vi "PH_ImageCalibrator.ProcCases.vi"(0 "i ref in":refnum<vi>, 1 "selector":string, 2 "data":T1, 3 "call cluster":T2={"Object"="", "Selector"="", "CallType"=enum."synchronous", "Async Object"="", "Async Selector"="", "Data Descriptor"="", "Data"=[], "Error #"=0, "Expire"=0}, 5 "error in":errorcluster) -> (14 "i ref out":refnum<vi>, 17 "answer cluster":T2={"Object"="", "Selector"="", "CallType"=enum."synchronous", "Async Object"="", "Async Selector"="", "Data Descriptor"="", "Data"=[], "Error #"=0, "Expire"=0}, 19 "error out":errorcluster)   [LabVIEW 2014, in "PH_ImageCalibrator.lvlib"]
doc: "This method is called by a process from within the default case in the event loop. The methods of a class that are linked to events will be called from THIS method. Add your code here."
uses:
  PH_ImageCalibrator.lvlib
  CSCore/CSSystem/CoreDefs/CoreDefs.call_type.ctl
  CSCore/BaseProcess/BaseProcess.descriptor string definition.ctl
  CSCore/CSSystem/CoreDefs/CoreDefs.rawDataType.ctl
  CSCore/CSSystem/CoreLib/CoreLib.string 2 byte array.vi
  CSCore/CSSystem/CoreLib/CoreLib.byte array 2 string.vi
  CSCore/BaseProcess/BaseProcess.lvlib
  CSCore/CSSystem/CoreLib/CoreLib.lvlib
  CSCore/BaseSM/BaseSM.lvlib
  PH_Img_BaseClass/PH_Img_BaseClass.lvlib
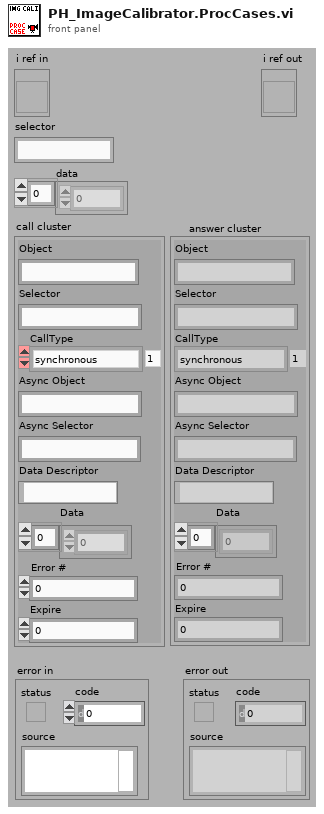
[diagram p1: front panel]
types:
  T1 = typedef "CoreDefs.rawDataType.ctl" = i8[]
  T2 = typedef "CoreDefs.call_type.ctl" = cluster{"Object":string, "Selector":string, "CallType":enum16{"simple", "synchronous", "asynchronous"}, "Async Object":string, "Async Selector":string, "Data Descriptor":T3, "Data":T1, "Error #":i32, "Expire":u32}
  T3 = typedef "BaseProcess.lvlib/BaseProcess.descriptor string definition.ctl" = string
  T4 = typedef "PH_ImageCalibrator.lvlib/PH_ImageCalibrator.i attribute.ctl" = cluster{"GUI Refs":cluster{"Available Cams":refnum<vi>, "OK":refnum<vi>, "Skip":refnum<vi>, "Repeat":refnum<vi>, "Cancel":refnum<vi>, "Length [mm]":refnum<vi>, "Energy [mJ]":refnum<vi>, "Dialog":refnum<vi>}, "Cam instances":string[], "Dark Pics":cluster{"#":i32, "BI taken":bool}, "Lin Cali":cluster{"Distance [Pixel]":dbl, "Distance [mm]":dbl, "Lin Cali Factor [mm/Pixel]":dbl}, "Energy Cali":cluster{"Pixelsum":dbl, "Energy [mJ]":dbl, "Energy Cali factor [mJ/Pixelsum]":dbl, "Underground subtracted?":bool, "#":i32}, "Images":cluster{"Background":T5, "Energy":T5}}
  T5 = typedef "IMAQ Image.ctl" = refnum<image>
  T6 = typedef "PH_Img_BaseClass.lvlib/PH_Img_BaseClass.i attribute.ctl" = cluster{"GUI Refs":T7, "Timeout Image [ms]":i32, "Default Periodic Period [ms]":i32, "Camera":cluster{"Instancename":string, "Notifier":refnum<notifier>}, "Palette":T8, "Cam Settings":cluster{"Cam ID":string, "Gain":dbl, "Brightness":dbl, "Shutter":dbl, "Cam Info Failure":bool, "Mode":i32}}
  T7 = typedef "PH_Img_BaseClass.lvlib/PH_Img_BaseClass.GUI Refs.ctl" = cluster{"Timeout":refnum<vi>, "Image":refnum<vi>, "Palette":refnum<vi>, "Timeout Set":refnum<vi>}
  T8 = typedef "PH_Img_BaseClass.lvlib/PH_Img_BaseClass.Palette.ctl" = i32
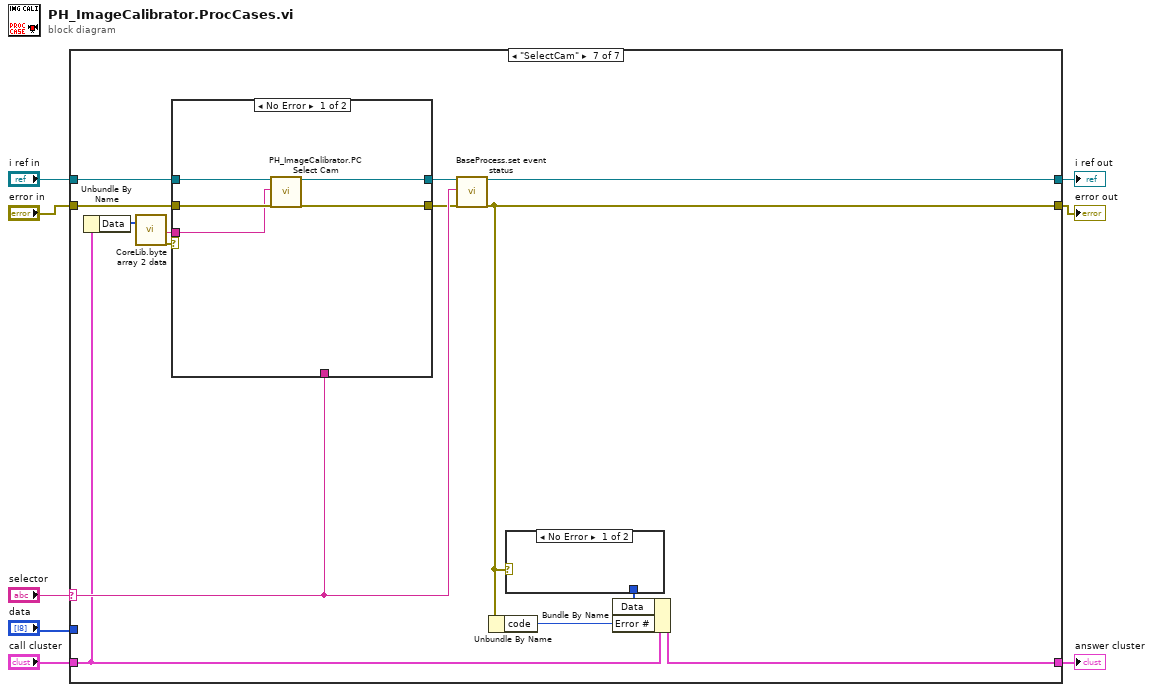
[diagram p0: block diagram]
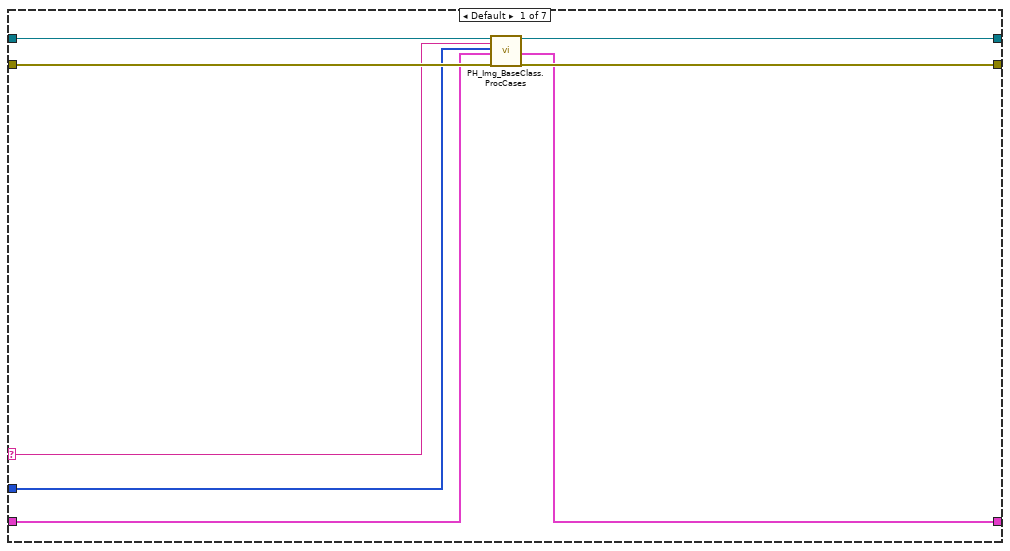
[diagram p2: hidden frame]
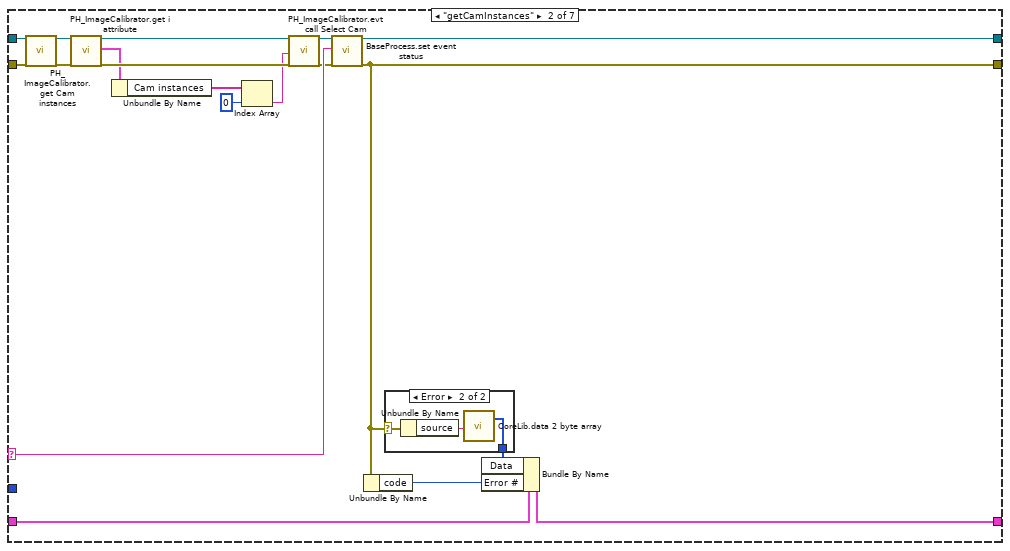
[diagram p3: hidden frame]
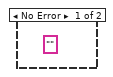
[diagram p4: hidden frame]
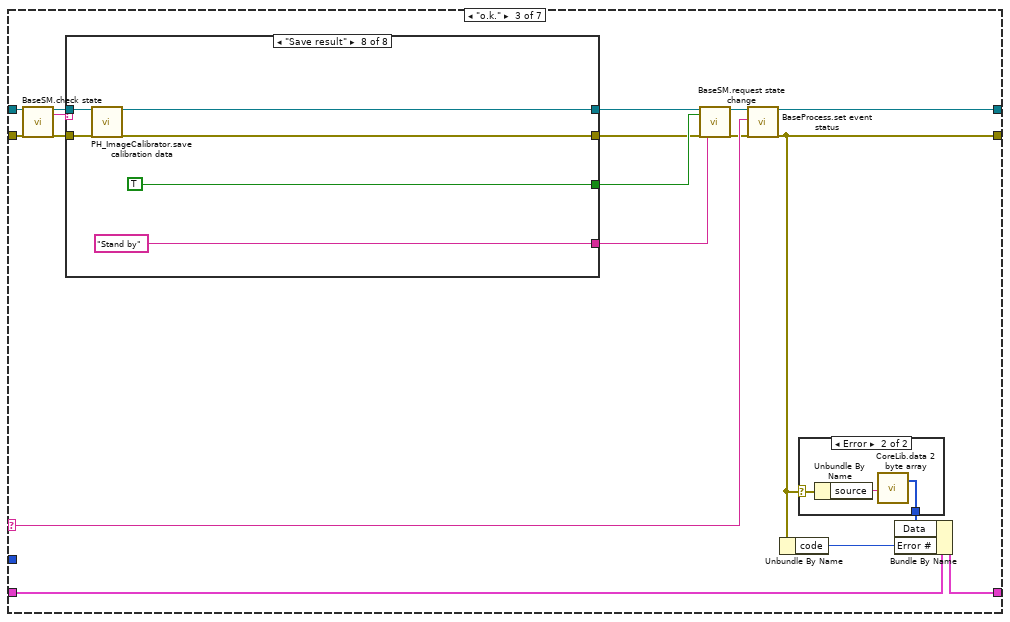
[diagram p5: hidden frame]
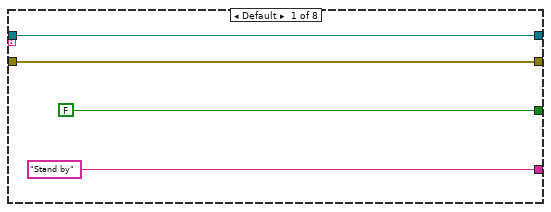
[diagram p6: hidden frame]
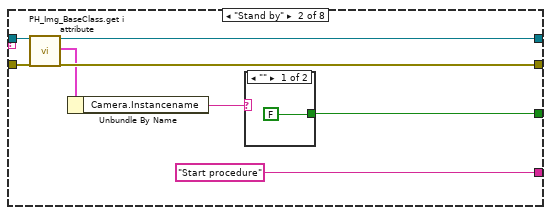
[diagram p7: hidden frame]
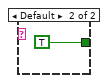
[diagram p8: hidden frame]
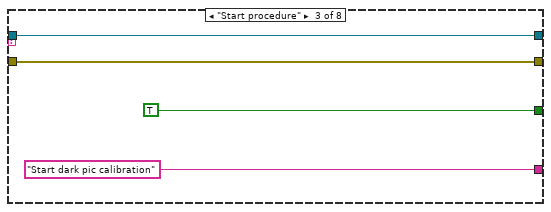
[diagram p9: hidden frame]
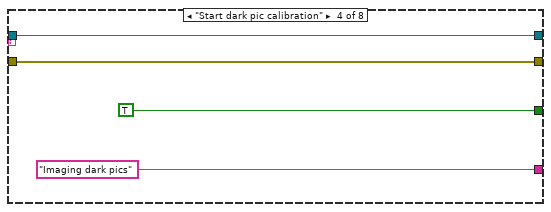
[diagram p10: hidden frame]
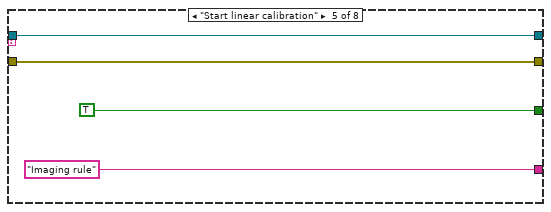
[diagram p11: hidden frame]
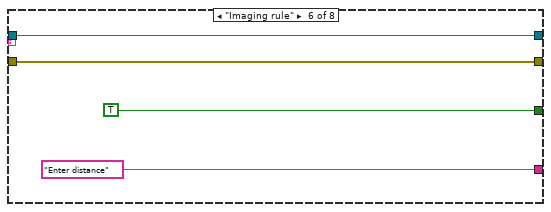
[diagram p12: hidden frame]
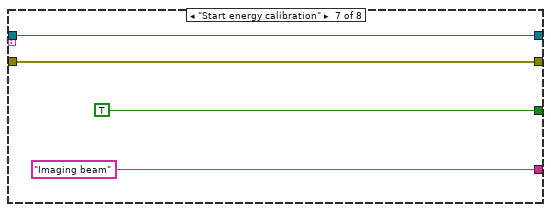
[diagram p13: hidden frame]
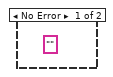
[diagram p14: hidden frame]
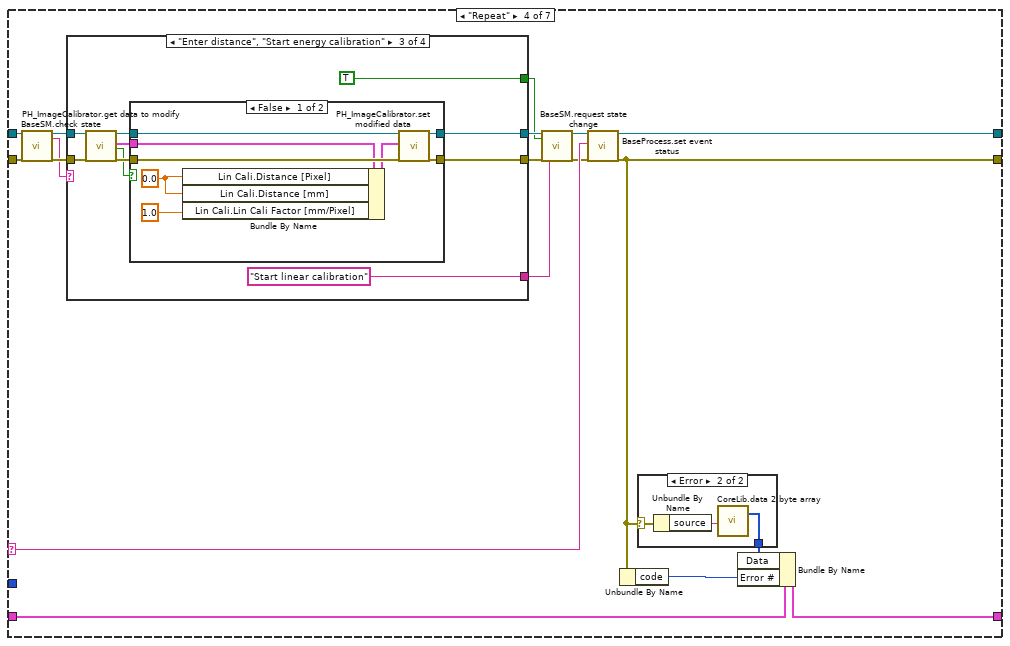
[diagram p15: hidden frame]
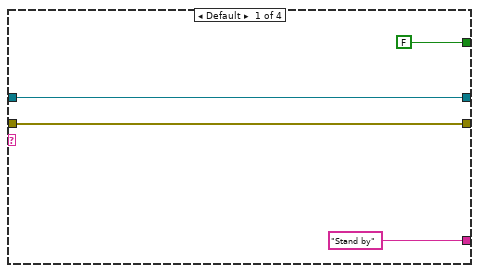
[diagram p16: hidden frame]
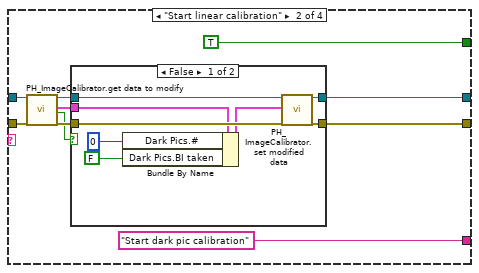
[diagram p17: hidden frame]
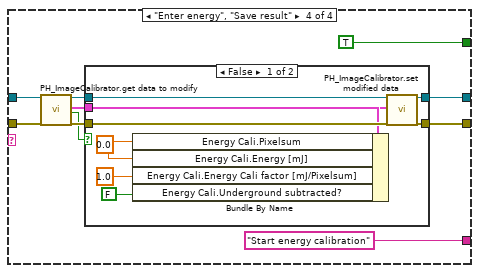
[diagram p20: hidden frame]
diagram:
  n1 = case shown="\"SelectCam\"" "selector" {
    selector: "selector" -> [w10 w31 w52 w113 w199 w286 w312]
    tunnel: "data" -> [w11 _ _ _ _ _ _]
    tunnel: "i ref in" -> [w9 w29 w50 w109 w195 w280 w310]
    tunnel: [w16 w30 w51 w112 w198 w285 w313] -> w4
    tunnel: "call cluster" -> [w12 w34 w55 w116 w202 w289 w311]
    tunnel: [w13 w33 w54 w115 w201 w288 w315] -> w7
    tunnel: "error in" -> [w15 w28 w49 w108 w194 w282 w308]
    tunnel: [w14 w32 w53 w114 w200 w287 w314] -> w3
    frame Default {
      n2 = call "PH_Img_BaseClass.ProcCases.vi"("i ref in"=w9, "selector"=w10, "Data"=w11, "call cluster"=w12, "error in (no error)"=w15) -> ("i ref out"=w16:refnum<vi>, "answer cluster"=w13:T2, "error out"=w14:errorcluster)  [unwired: 12 in]
    }
    frame "getCamInstances" {
      n3 = call "PH_ImageCalibrator.get Cam instances.vi"("i ref in"=w29, "error in"=w28) -> ("i ref out"=w27:refnum<vi>, "error out"=w24:errorcluster)  [unwired: 16 in]
      n4 = call "PH_ImageCalibrator.get i attribute.vi"("i ref in"=w27, "error in (no error)"=w24) -> ("i ref out"=w18:refnum<vi>, "i attribute"=w22:T4, "error out"=w25:errorcluster)  [unwired: 15 in]
      n5 = Unbundle By Name(w22) -> ("Cam instances"=w21:string[])
      n6 = Index Array(array=w21, index=0) -> (element=w19:string)
      n7 = call "PH_ImageCalibrator.evt call Select Cam.vi"("i ref in"=w18, "Cam"=w19, "error in"=w25) -> ("i ref out"=w26:refnum<vi>, "error out"=w23:errorcluster)  [unwired: 15 in]
      n8 = call "BaseProcess.set event status.vi"("i ref in"=w26, "EventStatus"=w31, "error in (no error)"=w23) -> ("i ref out"=w30:refnum<vi>, "error out"=w32:errorcluster)  [unwired: 14 in, 1 out]
      n9 = Unbundle By Name(w32) -> ("code"=w35:i32)
      n10 = case shown="Error" w32 {
        selector: w32 -> [_ w38]
        tunnel: [_ w36] -> w17
        frame No Error {
          (unwired) "" ("source")
        }
        frame Error {
          n11 = Unbundle By Name(w38) -> ("source"=w37:string)
          n12 = call-poly "CoreLib.data 2 byte array.vi"("string"=w37) -> ("byteArray out"=w36:T1)  [unwired: 18 in]
        }
      }
      n13 = Bundle By Name(cluster=w34, "Data"=w17, "Error #"=w35) -> (w33:T2)
    }
    frame "o.k." {
      n14 = call "BaseSM.check state.vi"("i ref in"=w50, "error in (no error)"=w49) -> ("i ref out"=w43:refnum<vi>, "actualState"=w44:string, "error out"=w41:errorcluster)  [unwired: 12 in, 3 out]
      n15 = case shown="\"Save result\"" w44 {
        tunnel: ["Stand by" ("requested state") "Start procedure" ("requested state") "Start dark pic calibration" ("requested state") "Imaging dark pics" ("requested state") "Imaging rule" ("requested state") "Enter distance" ("requested state") "Imaging beam" ("requested state") "Stand by" ("requested state")] -> w46
        tunnel: [FALSE ("change") w67 TRUE ("change") TRUE ("change") TRUE ("change") TRUE ("change") TRUE ("change") TRUE ("change")] -> w45
        tunnel: w43 -> [w58 w66 w72 w76 w80 w84 w87 w94]
        tunnel: [w58 w65 w72 w76 w80 w84 w87 w93] -> w42
        tunnel: w41 -> [w57 w64 w71 w75 w79 w83 w88 w92]
        tunnel: [w57 w63 w71 w75 w79 w83 w88 w91] -> w40
        frame Default {
        }
        frame "Stand by" {
          n16 = call "PH_Img_BaseClass.get i attribute.vi"("i ref in"=w66, "error in (no error)"=w64) -> ("i ref out"=w65:refnum<vi>, "i attribute"=w62:T6, "error out"=w63:errorcluster)  [unwired: 15 in]
          n17 = Unbundle By Name(w62) -> ("Camera.Instancename"=w61:string)
          n18 = case shown="\"\"" w61 {
            tunnel: [FALSE TRUE ("change")] -> w67
            frame "" {
            }
            frame Default {
            }
          }
        }
        frame "Start procedure" {
        }
        frame "Start dark pic calibration" {
        }
        frame "Start linear calibration" {
        }
        frame "Imaging rule" {
        }
        frame "Start energy calibration" {
        }
        frame "Save result" {
          n19 = call "PH_ImageCalibrator.save calibration data.vi"("i ref in"=w94, "error in (no error)"=w92) -> ("i ref out"=w93:refnum<vi>, "error out"=w91:errorcluster)  [unwired: 16 in]
        }
      }
      n20 = call "BaseSM.request state change.vi"("i ref in"=w42, "change"=w45, "error in (no error)"=w40, "requested state"=w46) -> ("i ref out"=w48:refnum<vi>, "error out"=w47:errorcluster)  [unwired: 12 in, 2 out]
      n21 = call "BaseProcess.set event status.vi"("i ref in"=w48, "EventStatus"=w52, "error in (no error)"=w47) -> ("i ref out"=w51:refnum<vi>, "error out"=w53:errorcluster)  [unwired: 14 in, 1 out]
      n22 = Unbundle By Name(w53) -> ("code"=w56:i32)
      n23 = case shown="Error" w53 {
        selector: w53 -> [_ w99]
        tunnel: [_ w98] -> w39
        frame No Error {
          (unwired) "" ("source")
        }
        frame Error {
          n24 = Unbundle By Name(w99) -> ("source"=w97:string)
          n25 = call-poly "CoreLib.data 2 byte array.vi"("string"=w97) -> ("byteArray out"=w98:T1)  [unwired: 18 in]
        }
      }
      n26 = Bundle By Name(cluster=w55, "Data"=w39, "Error #"=w56) -> (w54:T2)
    }
    frame "Repeat" {
      n27 = call "BaseSM.check state.vi"("i ref in"=w109, "error in (no error)"=w108) -> ("i ref out"=w111:refnum<vi>, "actualState"=w107:string, "error out"=w110:errorcluster)  [unwired: 12 in, 3 out]
      n28 = case shown="\"Enter distance\", \"Start energy calibration\"" w107 {
        tunnel: [w121 w125 w142 w162] -> w103
        tunnel: [w120 w124 w144 w164] -> w105
        tunnel: w111 -> [w121 w129 w143 w163]
        tunnel: w110 -> [w120 w128 w145 w165]
        tunnel: [FALSE TRUE TRUE TRUE] -> w102
        tunnel: ["Stand by" "Start dark pic calibration" "Start linear calibration" "Start energy calibration"] -> w101
        frame Default {
        }
        frame "Start linear calibration" {
          n29 = call "PH_ImageCalibrator.get data to modify.vi"("i ref in"=w129, "error in (no error)"=w128) -> ("i ref out"=w131:refnum<vi>, "i attribute"=w127:T4, "timed out"=w126:bool, "error out"=w130:errorcluster)  [unwired: 14 in]
          n30 = case shown="False" w126 {
            tunnel: w131 -> [w139 w141]
            tunnel: w130 -> [w138 w140]
            tunnel: [w137 w141] -> w125
            tunnel: [w136 w140] -> w124
            tunnel: w127 -> [w135 _]
            frame False {
              n31 = Bundle By Name(cluster=w135, "Dark Pics.#"=0, "Dark Pics.BI taken"=FALSE) -> (w134:T4)
              n32 = call "PH_ImageCalibrator.set modified data.vi"("i ref in"=w139, "i attribute"=w134, "error in (no error)"=w138) -> ("i ref out"=w137:refnum<vi>, "error out"=w136:errorcluster)  [unwired: 15 in]
            }
            frame True {
            }
          }
        }
        frame "Enter distance", "Start energy calibration" {
          n33 = call "PH_ImageCalibrator.get data to modify.vi"("i ref in"=w143, "error in (no error)"=w145) -> ("i ref out"=w149:refnum<vi>, "i attribute"=w147:T4, "timed out"=w146:bool, "error out"=w148:errorcluster)  [unwired: 14 in]
          n34 = case shown="False" w146 {
            tunnel: w149 -> [w159 w161]
            tunnel: w148 -> [w158 w160]
            tunnel: [w157 w161] -> w142
            tunnel: [w156 w160] -> w144
            tunnel: w147 -> [w155 _]
            frame False {
              w153 = 0.0 ("Lin Cali.Distance [Pixel]")
              n35 = Bundle By Name(cluster=w155, "Lin Cali.Distance [Pixel]"=w153, "Lin Cali.Distance [mm]"=w153, "Lin Cali.Lin Cali Factor [mm/Pixel]"=1.0) -> (w154:T4)
              n36 = call "PH_ImageCalibrator.set modified data.vi"("i ref in"=w159, "i attribute"=w154, "error in (no error)"=w158) -> ("i ref out"=w157:refnum<vi>, "error out"=w156:errorcluster)  [unwired: 15 in]
            }
            frame True {
            }
          }
        }
        frame "Enter energy", "Save result" {
          n37 = call "PH_ImageCalibrator.get data to modify.vi"("i ref in"=w163, "error in (no error)"=w165) -> ("i ref out"=w169:refnum<vi>, "i attribute"=w167:T4, "timed out"=w166:bool, "error out"=w168:errorcluster)  [unwired: 14 in]
          n38 = case shown="False" w166 {
            tunnel: w169 -> [w180 w182]
            tunnel: w168 -> [w179 w181]
            tunnel: [w178 w182] -> w162
            tunnel: [w177 w181] -> w164
            tunnel: w167 -> [w176 _]
            frame False {
              w174 = 0.0 ("Lin Cali.Distance [Pixel]")
              n39 = Bundle By Name(cluster=w176, "Energy Cali.Pixelsum"=w174, "Energy Cali.Energy [mJ]"=w174, "Energy Cali.Energy Cali factor [mJ/Pixelsum]"=1.0 ("Lin Cali.Lin Cali Factor [mm/Pixel]"), "Energy Cali.Underground subtracted?"=FALSE) -> (w175:T4)
              n40 = call "PH_ImageCalibrator.set modified data.vi"("i ref in"=w180, "i attribute"=w175, "error in (no error)"=w179) -> ("i ref out"=w178:refnum<vi>, "error out"=w177:errorcluster)  [unwired: 15 in]
            }
            frame True {
            }
          }
        }
      }
      n41 = call "BaseSM.request state change.vi"("i ref in"=w103, "change"=w102, "error in (no error)"=w105, "requested state"=w101) -> ("i ref out"=w104:refnum<vi>, "error out"=w106:errorcluster)  [unwired: 12 in, 2 out]
      n42 = call "BaseProcess.set event status.vi"("i ref in"=w104, "EventStatus"=w113, "error in (no error)"=w106) -> ("i ref out"=w112:refnum<vi>, "error out"=w114:errorcluster)  [unwired: 14 in, 1 out]
      n43 = Unbundle By Name(w114) -> ("code"=w117:i32)
      n44 = case shown="Error" w114 {
        selector: w114 -> [_ w185]
        tunnel: [_ w183] -> w100
        frame No Error {
          (unwired) "" ("source")
        }
        frame Error {
          n45 = Unbundle By Name(w185) -> ("source"=w184:string)
          n46 = call-poly "CoreLib.data 2 byte array.vi"("string"=w184) -> ("byteArray out"=w183:T1)  [unwired: 18 in]
        }
      }
      n47 = Bundle By Name(cluster=w116, "Data"=w100, "Error #"=w117) -> (w115:T2)
    }
    frame "Skip" {
      n48 = call "BaseSM.check state.vi"("i ref in"=w195, "error in (no error)"=w194) -> ("i ref out"=w197:refnum<vi>, "actualState"=w193:string, "error out"=w196:errorcluster)  [unwired: 12 in, 3 out]
      n49 = case shown="\"Enter distance\", \"Imaging rule\", \"Start linear calibration\"" w193 {
        tunnel: [w207 w209 w230 w254] -> w189
        tunnel: [w206 w208 w232 w253] -> w187
        tunnel: w197 -> [w207 w214 w236 w256]
        tunnel: w196 -> [w206 w215 w235 w255]
        tunnel: ["Stand by" ("requested state") "Start linear calibration" ("requested state") "Start energy calibration" ("requested state") "Save result" ("requested state")] -> w192
        tunnel: [FALSE TRUE TRUE TRUE] -> w191
        frame Default {
        }
        frame "Start dark pic calibration" {
          n50 = call "PH_ImageCalibrator.get data to modify.vi"("i ref in"=w214, "error in (no error)"=w215) -> ("i ref out"=w217:refnum<vi>, "i attribute"=w212:T4, "timed out"=w213:bool, "error out"=w216:errorcluster)  [unwired: 14 in]
          n51 = case shown="False" w213 {
            tunnel: w217 -> [w225 w227]
            tunnel: w216 -> [w224 w226]
            tunnel: [w223 w226] -> w208
            tunnel: [w222 w227] -> w209
            tunnel: w212 -> [w221 _]
            frame False {
              n52 = Bundle By Name(cluster=w221, "Dark Pics.#"=0, "Dark Pics.BI taken"=FALSE) -> (w220:T4)
              n53 = call "PH_ImageCalibrator.set modified data.vi"("i ref in"=w225, "i attribute"=w220, "error in (no error)"=w224) -> ("i ref out"=w222:refnum<vi>, "error out"=w223:errorcluster)  [unwired: 15 in]
            }
            frame True {
            }
          }
        }
        frame "Enter distance", "Imaging rule", "Start linear calibration" {
          w228 = u32 0 items=["Zoom Tool"=8, "Selection Tool"=0, "Pan Tool"=9, "Point Tool"=1, "Line Tool"=2, "Rectangle Tool"=3, "Rotated Rectangle Tool"=12, "Polyline Tool"=10, "Polygon Tool"=5, "Freehand Tool"=11, "Closed Freehand Tool"=6, "Ellipse Tool"=4, "Annulus Tool"=7] ("ROI Tool")
          n54 = call "PH_ImageCalibrator.get data to modify.vi"("i ref in"=w236, "error in (no error)"=w235) -> ("i ref out"=w240:refnum<vi>, "i attribute"=w237:T4, "timed out"=w238:bool, "error out"=w239:errorcluster)  [unwired: 14 in]
          n55 = case shown="False" w238 {
            tunnel: w240 -> [w248 w250]
            tunnel: w239 -> [w247 w249]
            tunnel: [w246 w249] -> w231
            tunnel: [w245 w250] -> w229
            tunnel: w237 -> [w244 _]
            frame False {
              w242 = 0.0 ("Lin Cali.Distance [Pixel]")
              n56 = Bundle By Name(cluster=w244, "Lin Cali.Distance [Pixel]"=w242, "Lin Cali.Distance [mm]"=w242, "Lin Cali.Lin Cali Factor [mm/Pixel]"=1.0) -> (w243:T4)
              n57 = call "PH_ImageCalibrator.set modified data.vi"("i ref in"=w248, "i attribute"=w243, "error in (no error)"=w247) -> ("i ref out"=w245:refnum<vi>, "error out"=w246:errorcluster)  [unwired: 15 in]
            }
            frame True {
            }
          }
          n58 = call "PH_ImageCalibrator.Set Image ROI.vi"("i ref in"=w229, "ROI Tool"=w228, "error in"=w231) -> ("i ref out"=w230:refnum<vi>, "error out"=w232:errorcluster)  [unwired: 15 in]
        }
        frame "Enter energy", "Start energy calibration" {
          n59 = call "PH_ImageCalibrator.get data to modify.vi"("i ref in"=w256, "error in (no error)"=w255) -> ("i ref out"=w260:refnum<vi>, "i attribute"=w257:T4, "timed out"=w258:bool, "error out"=w259:errorcluster)  [unwired: 14 in]
          n60 = case shown="False" w258 {
            tunnel: w260 -> [w269 w271]
            tunnel: w259 -> [w268 w270]
            tunnel: [w267 w270] -> w253
            tunnel: [w266 w271] -> w254
            tunnel: w257 -> [w265 _]
            frame False {
              w263 = 0.0 ("Lin Cali.Distance [Pixel]")
              n61 = Bundle By Name(cluster=w265, "Energy Cali.Pixelsum"=w263, "Energy Cali.Energy [mJ]"=w263, "Energy Cali.Energy Cali factor [mJ/Pixelsum]"=1.0 ("Lin Cali.Lin Cali Factor [mm/Pixel]"), "Energy Cali.Underground subtracted?"=FALSE) -> (w264:T4)
              n62 = call "PH_ImageCalibrator.set modified data.vi"("i ref in"=w269, "i attribute"=w264, "error in (no error)"=w268) -> ("i ref out"=w266:refnum<vi>, "error out"=w267:errorcluster)  [unwired: 15 in]
            }
            frame True {
            }
          }
        }
      }
      n63 = call "BaseSM.request state change.vi"("i ref in"=w189, "change"=w191, "error in (no error)"=w187, "requested state"=w192) -> ("i ref out"=w190:refnum<vi>, "error out"=w188:errorcluster)  [unwired: 12 in, 2 out]
      n64 = call "BaseProcess.set event status.vi"("i ref in"=w190, "EventStatus"=w199, "error in (no error)"=w188) -> ("i ref out"=w198:refnum<vi>, "error out"=w200:errorcluster)  [unwired: 14 in, 1 out]
      n65 = Unbundle By Name(w200) -> ("code"=w203:i32)
      n66 = case shown="Error" w200 {
        selector: w200 -> [_ w274]
        tunnel: [_ w272] -> w186
        frame No Error {
          (unwired) "" ("source")
        }
        frame Error {
          n67 = Unbundle By Name(w274) -> ("source"=w273:string)
          n68 = call-poly "CoreLib.data 2 byte array.vi"("string"=w273) -> ("byteArray out"=w272:T1)  [unwired: 18 in]
        }
      }
      n69 = Bundle By Name(cluster=w202, "Data"=w186, "Error #"=w203) -> (w201:T2)
    }
    frame "Cancel" {
      w276 = "Stand by" ("y")
      n70 = call "BaseSM.check state.vi"("i ref in"=w280, "error in (no error)"=w282) -> ("i ref out"=w279:refnum<vi>, "actualState"=w277:string, "error out"=w281:errorcluster)  [unwired: 12 in, 3 out]
      n71 = Equal?(x=w277, y=w276) -> (x = y?=w278:bool)
      n72 = case shown="False" w278 {
        tunnel: [w297 w299] -> w284
        tunnel: [w296 w298] -> w283
        tunnel: w281 -> [w295 w298]
        tunnel: w279 -> [w293 w299]
        tunnel: w276 -> [w291 _]
        frame False {
          n73 = call "BaseSM.request state change.vi"("i ref in"=w293, "error in (no error)"=w295, "requested state"=w291) -> ("i ref out"=w292:refnum<vi>, "error out"=w294:errorcluster)  [unwired: 13 in, 2 out]
          n74 = call "PH_ImageCalibrator.reset Attributes.vi"("i ref in"=w292, "error in (no error)"=w294) -> ("i ref out"=w297:refnum<vi>, "error out"=w296:errorcluster)  [unwired: 16 in]
        }
        frame True {
        }
      }
      n75 = call "BaseProcess.set event status.vi"("i ref in"=w284, "EventStatus"=w286, "error in (no error)"=w283) -> ("i ref out"=w285:refnum<vi>, "error out"=w287:errorcluster)  [unwired: 14 in, 1 out]
      n76 = Unbundle By Name(w287) -> ("code"=w290:i32)
      n77 = case shown="Error" w287 {
        selector: w287 -> [_ w302]
        tunnel: [_ w300] -> w275
        frame No Error {
          (unwired) "" ("source")
        }
        frame Error {
          n78 = Unbundle By Name(w302) -> ("source"=w301:string)
          n79 = call-poly "CoreLib.data 2 byte array.vi"("string"=w301) -> ("byteArray out"=w300:T1)  [unwired: 18 in]
        }
      }
      n80 = Bundle By Name(cluster=w289, "Data"=w275, "Error #"=w290) -> (w288:T2)
    }
    frame "SelectCam" {
      n81 = Unbundle By Name(w311) -> ("Data"=w306:T1)
      n82 = call-poly "CoreLib.byte array 2 data.vi"("byteArray"=w306) -> ("string"=w305:string, "error out"=w304:errorcluster)  [unwired: 16 in, 1 out]
      n83 = case shown="No Error" w304 {
        tunnel: w310 -> [w321 w323]
        tunnel: [w317 w323] -> w309
        tunnel: w308 -> [w320 w325]
        tunnel: [w318 w324] -> w307
        tunnel: w312 -> [_ w322]
        tunnel: w305 -> [w319 _]
        frame No Error {
          n84 = call "PH_ImageCalibrator.PC Select Cam.vi"("VI in"=w321, "Source"=w319, "error in (no error)"=w320) -> ("VI out"=w317:refnum<vi>, "error out"=w318:errorcluster)  [unwired: 15 in]
        }
        frame Error {
          n85 = call "CoreLib.set data type mismatch.vi"("error in (no error)"=w325, "error source"=w322) -> ("error out"=w324:errorcluster)  [unwired: 17 in]
        }
      }
      n86 = call "BaseProcess.set event status.vi"("i ref in"=w309, "EventStatus"=w312, "error in (no error)"=w307) -> ("i ref out"=w313:refnum<vi>, "error out"=w314:errorcluster)  [unwired: 14 in, 1 out]
      n87 = Unbundle By Name(w314) -> ("code"=w316:i32)
      n88 = case shown="No Error" w314 {
        selector: w314 -> [_ w328]
        tunnel: [_ w326] -> w303
        frame No Error {
        }
        frame Error {
          n89 = Unbundle By Name(w328) -> ("source"=w327:string)
          n90 = call-poly "CoreLib.data 2 byte array.vi"("string"=w327) -> ("byteArray out"=w326:T1)  [unwired: 18 in]
        }
      }
      n91 = Bundle By Name(cluster=w311, "Data"=w303, "Error #"=w316) -> (w315:T2)
    }
  }
  "answer cluster" <- w7
  "i ref out" <- w4
  "error out" <- w3
